vi "CSM - Debug Console - DebugTool.vi"   [LabVIEW 2017]
doc: "New version of the CSM Debug Console, you can use this tool:\n1. Select an existing CSM instance, open the front panel and block diagram.\n2. Scan the API interfaces of existing CSM instances, including the API list of Python CSM modules. The API list is auto-filled, and APIs that are not predefined can also be called.\n3. Select an API interface, call synchronously or asynchronously, view the return value.\n4. View the overall program's running log.\n5. Run Scripts."
uses:
  _debugConsole/CSM - Debug Console 2.vi
  _debugConsole/DebugConsole.lvlib
  _ui/csm-ui-support.lvlib
types:
  T1 = enum32{"Bad", "Idle", "Run top level", "Running"}
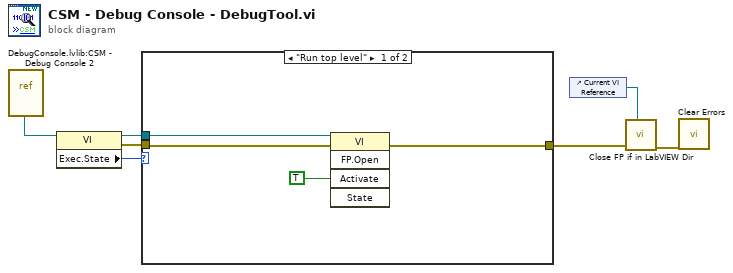
[diagram p0: block diagram]
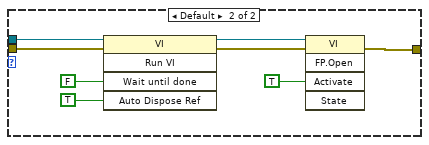
[diagram p2: hidden frame]
diagram:
  n1 = vi-ref "DebugConsole.lvlib:CSM - Debug Console 2.vi"() -> (w7:refnum<vi>)
  n2 = property class="VI"(reference=w7) -> (reference out=w5:refnum<vi>, error out=w4:errorcluster, "Exec.State"=w6:T1)  [unwired: 1 in]
  n3 = case shown="\"Run top level\"" w6 {
    tunnel: w5 -> [w10 w19]
    tunnel: w4 -> [w11 w18]
    tunnel: [w8 w12] -> w1
    frame "Run top level" {
      n4 = invoke class="VI" method="FP.Open"(reference=w10, error in=w11, "Activate"=TRUE ("Activate?")) -> (error out=w8:errorcluster)  [unwired: 2 in, 4 out]
    }
    frame Default {
      n5 = invoke class="VI" method="Run VI"(reference=w19, error in=w18, "Wait until done"=FALSE ("Wait Until Done"), "Auto Dispose Ref"=TRUE ("Auto Dispose Reference")) -> (reference out=w15:refnum<vi>, error out=w14:errorcluster)  [unwired: 1 in, 3 out]
      n6 = invoke class="VI" method="FP.Open"(reference=w15, error in=w14, "Activate"=TRUE ("Activate?")) -> (error out=w12:errorcluster)  [unwired: 2 in, 4 out]
    }
  }
  n7 = control-ref of="Current VI Reference"() -> (w2:refnum<vi>)
  n8 = call "Close FP if in LabVIEW Dir.vi"("VI Refnum"=w2, "Error in"=w1) -> ("Error out"=w3:errorcluster)  [unwired: 9 in]
  n9 = call <vilib>:"Clear Errors.vi"("error in (no error)"=w3) -> ()  [unwired: 5 in, 2 out]
